vi "initialise.vi"(0 "error in (no error)":errorcluster) -> (7 "error out":errorcluster, 8 "configuration":T1, 9 "network streaming queues":T2, 10 "FPGA VI Reference Out":refnum<k20>)   [LabVIEW 2010]
uses:
  network_streaming_queues_cluster.ctl
  scan_specification_cluster.ctl
  config_data_cluster.ctl
  <vilib>/userDefined/High Color/nirio_resource_hc.ctl
  <vilib>/rvi/interface/nirviOpenFPGA/nirviOpenFPGA.xnode
  FPGA Bitfiles/main.lvbitx
  <vilib>/rvi/ClientSDK/nirviWhatTheDeviceIsDoing.ctl
  <vilib>/rvi/interface/nirviMethod/nirviMethod.xnode
  <vilib>/rvi/interface/nirviReadWriteControl/nirviReadWriteControl.xnode
  <vilib>/rvi/interface/common/niFpgaNodeNameForErrorReporting.ctl
  <vilib>/rvi/errors/niLvFpgaWhatHappensToTopLevelVI.ctl
  <vilib>/FPGAPlugInAG/PXI-7813R/niLvFpga_Open_PXI-7813R.vi
  <vilib>/rvi/interface/common/dynamic/niFpgaDynamicAddResources.vi
  <vilib>/FPGAPlugInAG/Dynamic/niLvFpga_Reset_Dynamic.vi
  <vilib>/Utility/error.llb/Error Cluster From Error Code.vi
  <vilib>/rvi/errors/niLvFpgaAdjustHostInterfaceError.vi
  NiFpgaLv.dll
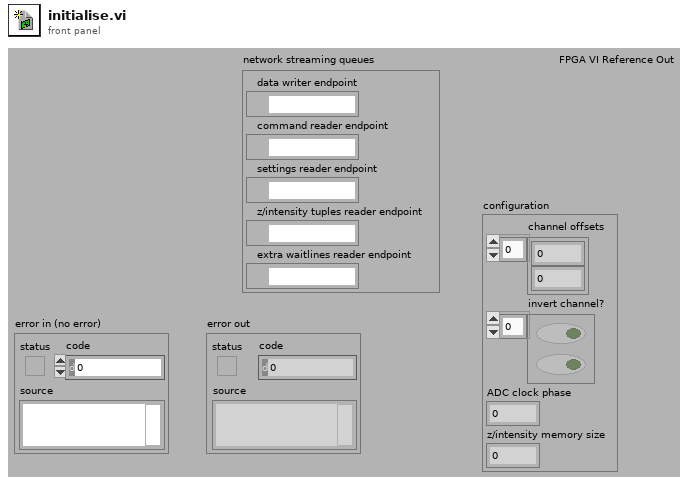
[diagram p1: front panel]
types:
  T1 = typedef "config_data_cluster.ctl" = cluster{"channel offsets":u32[], "invert channel?":bool[], "ADC clock phase":i32, "z/intensity memory size":i32}
  T2 = typedef "network_streaming_queues_cluster.ctl" = cluster{"data writer endpoint":refnum<k21>, "command reader endpoint":refnum<k21>, "settings reader endpoint":refnum<k21>, "z/intensity tuples reader endpoint":refnum<k21>, "extra waitlines reader endpoint":refnum<k21>}
  T3 = typedef "scan_specification_cluster.ctl" = cluster{"x amplitude":u16, "x resolution (pixels)":u16, "x offset fly-forward (iterations)":u16, "x offset fly-back (iterations)":u16, "y resolution (nr. of lines)":u16, "y step size":u16, "iterations per pixel":u16, "number of frames":i32, "y offset (pixels)":u16, "number of y-brake lines  (before y-fly-back)":u16, "number y-brake lines (after y-fly-back)":u16, "number of y-fly-back steps":u16, "lines per z step":u16, "number of z/intensity tuples":u16, "number of repetitions (volumes or planes)":i32}
  T4 = cluster{"channel 0":u32, "channel 1":u32, "channel 2":u32, "channel 3":u32}
  T5 = typedef "nirio_resource_hc.ctl" = tag
  T6 = typedef "niFpgaNodeNameForErrorReporting.ctl" = enum16{"Open FPGA VI Reference", "Read/Write Control", "Invoke Method: Abort", "Invoke Method: Acknowledge IRQ", "Invoke Method: Download", "Invoke Method: FIFO.Configure", "Invoke Method: FIFO.Read", "Invoke Method: FIFO.Start", "Invoke Method: FIFO.Stop", "Invoke Method: FIFO.Write", "Invoke Method: Reset", "Invoke Method: Run", "Invoke Method: Wait on IRQ", "Close FPGA VI Reference"}
  T7 = typedef "niLvFpgaWhatHappensToTopLevelVI.ctl" = enum16{"top level VI scripted behind XNode", "top level VI inlined behind XNode"}
  T8 = typedef "nirviWhatTheDeviceIsDoing.ctl" = enum32{"nothing", "something other than LabVIEW FPGA", "FPGA interface", "interactive", "emulation"}
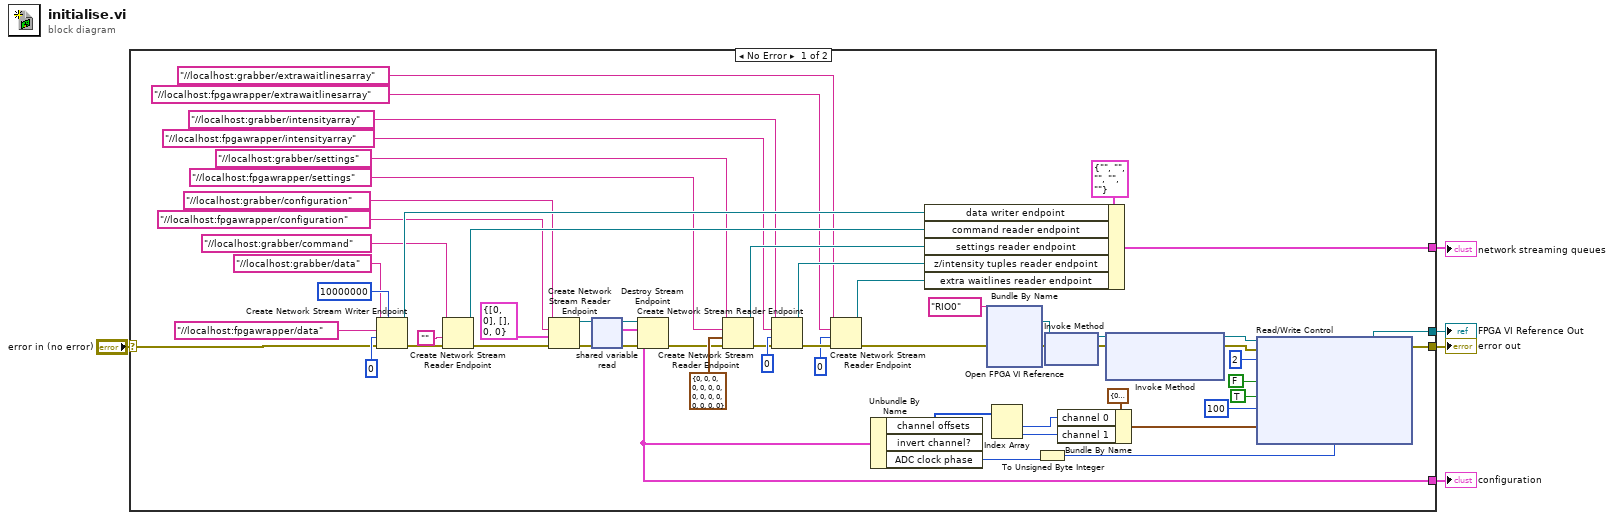
[diagram p0: block diagram]
diagram:
  n1 = case shown="No Error" "error in (no error)" {
    selector: "error in (no error)" -> [w32 w314]
    tunnel: [w31 w314] -> w4
    tunnel: [w53 _] -> w1
    tunnel: [w45 _] -> w3
    tunnel: [w26 _] -> w2
    frame No Error {
      n2 = Create Network Stream Writer Endpoint(7:10000000 ("writer buffer size"), 8:w32, 9:u32 0, 10:"//localhost:fpgawrapper/data" ("reader url"), 11:"//localhost:grabber/data" ("writer name")) -> (0:w42:errorcluster, 3:w46:refnum<k21>)  [unwired: 1 in]
      n3 = Create Network Stream Reader Endpoint(8:w42, 9:"", 11:"//localhost:grabber/command" ("reader name")) -> (0:w12:errorcluster, 3:w41:refnum<k21>)  [unwired: 3 in]
      n4 = Create Network Stream Reader Endpoint(8:w12, 9:T1 {"channel offsets"=[0, 0], "invert channel?"=[], "ADC clock phase"=0, "z/intensity memory size"=0} ("configuration"), 10:"//localhost:fpgawrapper/configuration" ("writer name"), 11:"//localhost:grabber/configuration" ("reader name")) -> (0:w36:errorcluster, 3:w35:refnum<k21>)  [unwired: 2 in]
      n5 = shared-variable-read(w35, w36) -> (w34:refnum<k21>, w37:errorcluster, w26:T1)  [unwired: 1 in, 1 out]
      n6 = Destroy Stream Endpoint(8:w37, 11:w34) -> (0:w14:errorcluster)
      n7 = Create Network Stream Reader Endpoint(8:w14, 9:T3 {"x amplitude"=0, "x resolution (pixels)"=0, "x offset fly-forward (iterations)"=0, "x offset fly-back (iterations)"=0, "y resolution (nr. of lines)"=0, "y step size"=0, "iterations per pixel"=0, "number of frames"=0, "y offset (pixels)"=0, "number of y-brake lines  (before y-fly-back)"=0, "number y-brake lines (after y-fly-back)"=0, "number of y-fly-back steps"=0, "lines per z step"=0, "number of z/intensity tuples"=0, "number of repetitions (volumes or planes)"=0} ("scan specification"), 10:"//localhost:fpgawrapper/settings" ("writer name"), 11:"//localhost:grabber/settings" ("reader name")) -> (0:w13:errorcluster, 3:w19:refnum<k21>)  [unwired: 2 in]
      n8 = Create Network Stream Reader Endpoint(8:w13, 9:u32 0, 10:"//localhost:fpgawrapper/intensityarray" ("writer name"), 11:"//localhost:grabber/intensityarray" ("reader name")) -> (0:w11:errorcluster, 3:w15:refnum<k21>)  [unwired: 2 in]
      n9 = Create Network Stream Reader Endpoint(8:w11, 9:u32 0, 10:"//localhost:fpgawrapper/extrawaitlinesarray" ("writer name"), 11:"//localhost:grabber/extrawaitlinesarray" ("reader name")) -> (0:w10:errorcluster, 3:w6:refnum<k21>)  [unwired: 2 in]
      n10 = Unbundle By Name(w26) -> ("channel offsets"=w33:u32[], "ADC clock phase"=w24:i32)  [unwired: 1 out]
      n11 = Bundle By Name(cluster=T2 {"data writer endpoint"="", "command reader endpoint"="", "settings reader endpoint"="", "z/intensity tuples reader endpoint"="", "extra waitlines reader endpoint"=""} ("network streaming queues"), "data writer endpoint"=w46, "command reader endpoint"=w41, "settings reader endpoint"=w19, "z/intensity tuples reader endpoint"=w15, "extra waitlines reader endpoint"=w6) -> (w45:T2)
      n12 = xnode "Open FPGA VI Reference"("error in"=w10, "resource name"=T5 "RIO0") -> ("FPGA VI Reference Out"=w55:refnum<k20>, "error out"=w56:errorcluster)
      n13 = Index Array(array=w33) -> (element #1=w28:u32, element #2=w27:u32)  [unwired: 2 in]
      n14 = To Unsigned Byte Integer(number=w24) -> (unsigned 8bit integer=w23:u8)
      n15 = xnode "Invoke Method"("FPGA VI Reference In"=w55, "error in"=w56) -> ("FPGA VI Reference Out"=w59:refnum<k20>, "error out"=w58:errorcluster)
      n16 = Bundle By Name(cluster=T4 {"channel 0"=0, "channel 1"=0, "channel 2"=0, "channel 3"=0} ("channel offsets"), "channel 0"=w28, "channel 1"=w27) -> (w29:T4)
      n17 = xnode "Invoke Method"("FPGA VI Reference In"=w59, "error in"=w58) -> ("FPGA VI Reference Out"=w61:refnum<k20>, "error out"=w60:errorcluster)  [unwired: 1 out]
      n18 = xnode "Read/Write Control"("FPGA VI Reference In"=w61, "error in"=w60, "converter box version"=i16 2, "FIFO overflow"=FALSE, "enable fly-back reversion?"=TRUE, "sync minimum high"=i16 100, "channel offsets"=w29, "ADC clock phase"=w23) -> ("FPGA VI Reference Out"=w53:refnum<k20>, "error out"=w31:errorcluster)
    }
    frame Error {
    }
  }
  "error out" <- w4
  "network streaming queues" <- w3
  "configuration" <- w2
  "FPGA VI Reference Out" <- w1
